vi "main.vi"() -> ()   [LabVIEW 2016]
uses:
  Base/Maze/Maze.lvclass
panel:
  out "new picture":picture
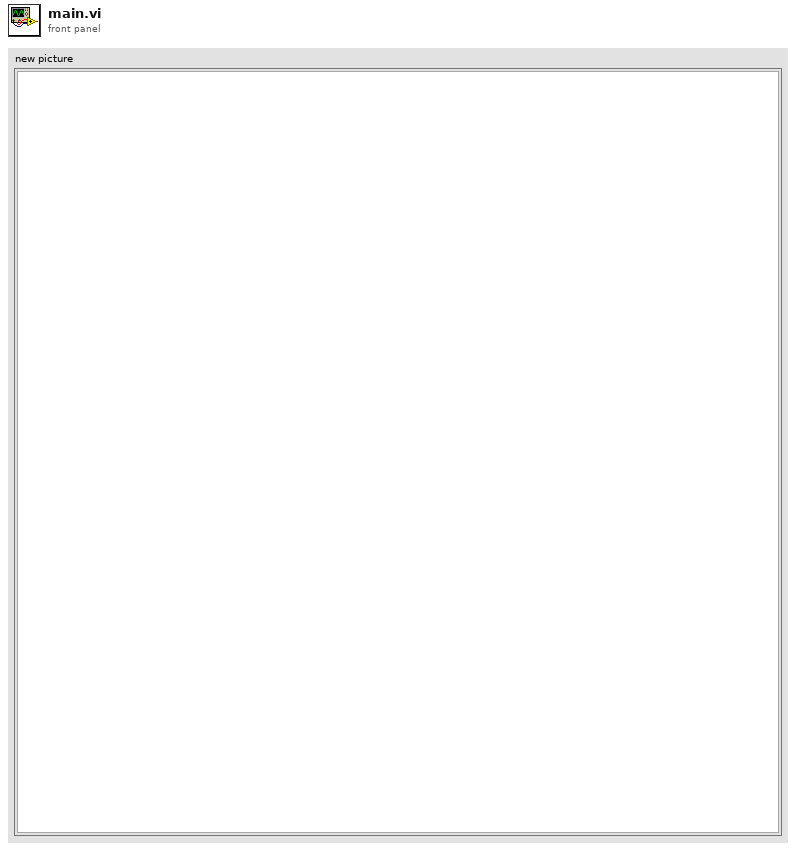
[diagram p1: front panel]
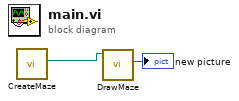
[diagram p0: block diagram]
diagram:
  n1 = call "CreateMaze.vi"() -> ("Maze*"=w2:refnum<data-value>)  [unwired: 10 in, 1 out]
  n2 = call "DrawMaze.vi"("Maze*"=w2) -> ("new picture"=→"new picture":picture)  [unwired: 9 in, 1 out]
